vi "Act On Test.vi"(6 "Report Action":T1, 8 "error in (no error)":errorcluster, 9 "Values":variant[](array[variant]), 10 "Parameters":string[](array[string]), 11 "Report in":refnum<class "Report.lvclass">) -> (0 "error out":errorcluster, 3 "Report out":refnum<class "Report.lvclass">)   [LabVIEW 2023, in "Report.lvlib" / "Report.lvclass"]
uses:
  Report.lvclass
  Custom Controls/Report Action.ctl
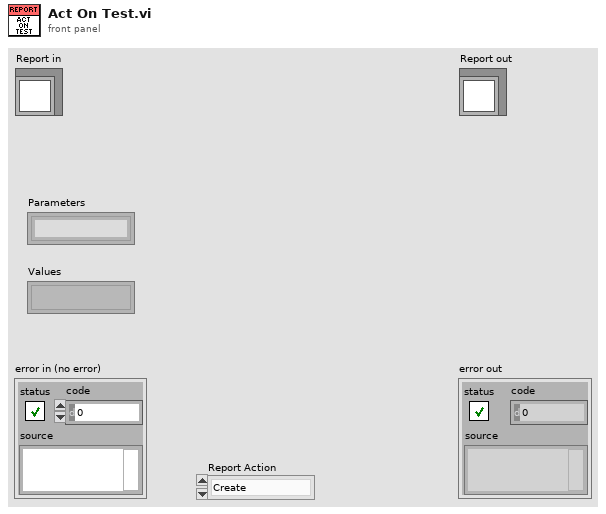
[diagram p1: front panel]
types:
  T1 = typedef "Report.lvlib/Report.lvclass/Report Action.ctl" = enum16{"Create", "Append", "Destroy"}
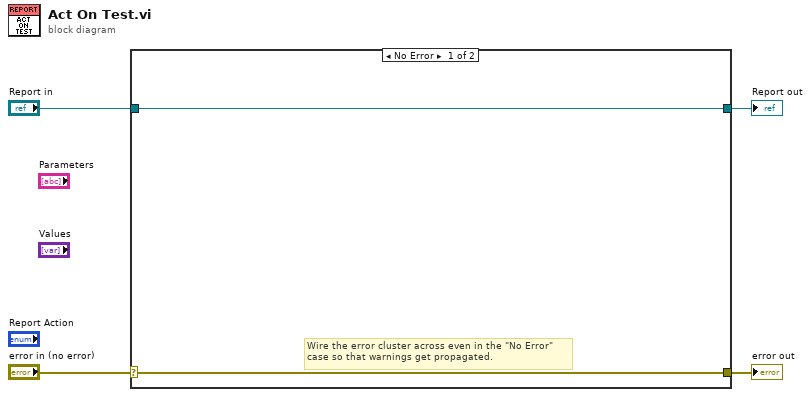
[diagram p0: block diagram]
diagram:
  n1 = case shown="No Error" "error in (no error)" {
    selector: "error in (no error)" -> [w5 w8]
    tunnel: [w5 w8] -> w3
    tunnel: [w6 w7] -> w1
    tunnel: "Report in" -> [w6 w7]
    frame No Error {
      # "Wire the error cluster across even in the \"No Error\"\ncase so that warnings get propagated."
    }
    frame Error {
    }
  }
  "error out" <- w3
  "Report out" <- w1
